vi "avg8_32bit.vi"(10 "Input":i32) -> (2 "Output":i32)   [LabVIEW 2011, in "kevLib2011.lvlib"]
uses:
  kevLib2011.lvlib
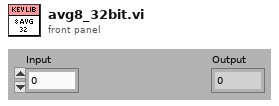
[diagram p1: front panel]
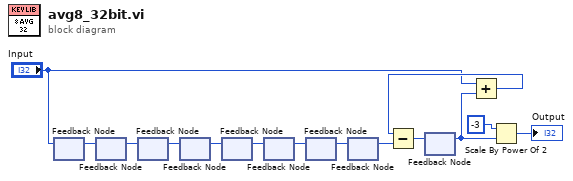
[diagram p0: block diagram]
diagram:
  n1 = feedback-in #1("Input") -> ()
  n2 = feedback #1() -> (w14:i32)  [unwired: 1 in]
  n3 = feedback-in #2(w14) -> ()
  n4 = feedback #2() -> (w13:i32)  [unwired: 1 in]
  n5 = feedback-in #3(w13) -> ()
  n6 = feedback #3() -> (w12:i32)  [unwired: 1 in]
  n7 = feedback-in #4(w12) -> ()
  n8 = feedback #4() -> (w11:i32)  [unwired: 1 in]
  n9 = feedback-in #5(w11) -> ()
  n10 = feedback #5() -> (w10:i32)  [unwired: 1 in]
  n11 = feedback-in #6(w10) -> ()
  n12 = feedback #6() -> (w9:i32)  [unwired: 1 in]
  n13 = feedback-in #7(w9) -> ()
  n14 = feedback #7() -> (w4:i32)  [unwired: 1 in]
  n15 = feedback-in #8(w4) -> ()
  n16 = feedback #8() -> (w3:i32)  [unwired: 1 in]
  n17 = feedback #9() -> (w6:i32)  [unwired: 1 in]
  n18 = Add(x="Input", y=w6) -> (x+y=w8:i32)
  n19 = Subtract(x=w8, y=w3) -> (x-y=w7:i32)
  n20 = feedback-in #9(w7) -> ()
  n21 = Scale By Power Of 2(n=-3, x=w6) -> (x*2^n=→"Output":i32)
